vi "DemoSubClass2_Create.vi"(0 "reference in":refnum<class "DemoSubClass2.lvclass">, 5 "error in (no error)":errorcluster) -> (14 "reference out":refnum<class "DemoSubClass2.lvclass">, 19 "error out":errorcluster)   [LabVIEW 2020, in "DemoSubClass2.lvclass"]
uses:
  DemoSubClass2.lvclass
  C:/Program Files (x86)/National Instruments/LabVIEW 2020/vi.lib/addons/_AddQ/G#Object/G#Object.lvclass
  C:/Program Files (x86)/National Instruments/LabVIEW 2020/examples/AddQ/G#/Polymorphism/DemoClass1_class/DemoClass1.lvclass
  DemoClass1_class/DemoClass1.lvclass
  vi.lib/addons/_AddQ/G#Object/G#Object.lvclass
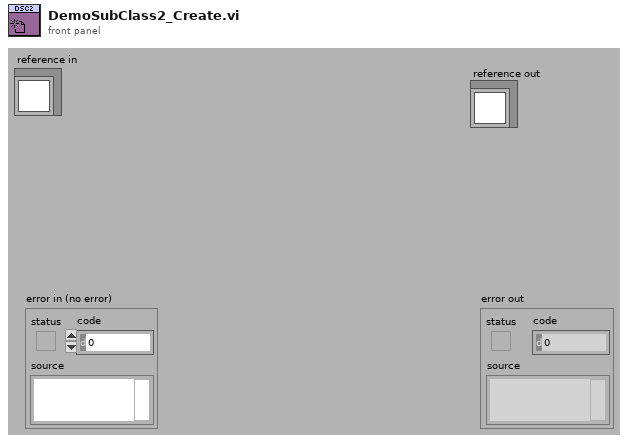
[diagram p1: front panel]
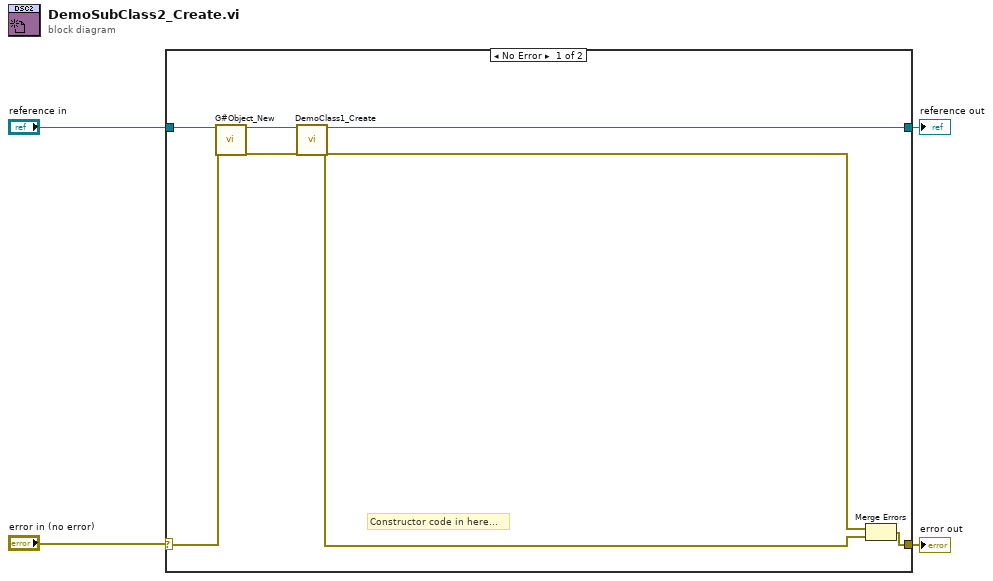
[diagram p0: block diagram]
diagram:
  n1 = case shown="No Error" "error in (no error)" {
    selector: "error in (no error)" -> [w11 w13]
    tunnel: [w8 w13] -> w3
    tunnel: [w5 w12] -> w2
    tunnel: "reference in" -> [w7 w12]
    frame No Error {
      # "Constructor code in here..."
      n2 = call "G#Object_New.vi"("reference in"=w7, "error in (no error)"=w11) -> ("reference out"=w9:refnum<class "DemoSubClass2.lvclass">, "error out"=w10:errorcluster)  [unwired: 15 in, 1 out]
      n3 = call "DemoClass1_Create.vi"("reference in"=w9, "error in (no error)"=w10) -> ("reference out"=w5:refnum<class "DemoSubClass2.lvclass">, "error out"=w6:errorcluster)  [unwired: 16 out]
      n4 = Merge Errors(w6, w6) -> (w8:errorcluster)
    }
    frame Error {
    }
  }
  "error out" <- w3
  "reference out" <- w2
